vi "PopulateNist.vi"(11 "Path":path=path "") -> (3 "Array":string[](array[string]))   [LabVIEW 2014]
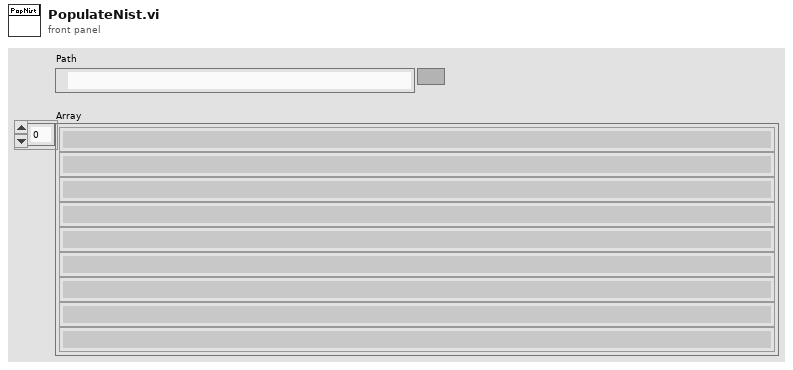
[diagram p1: front panel]
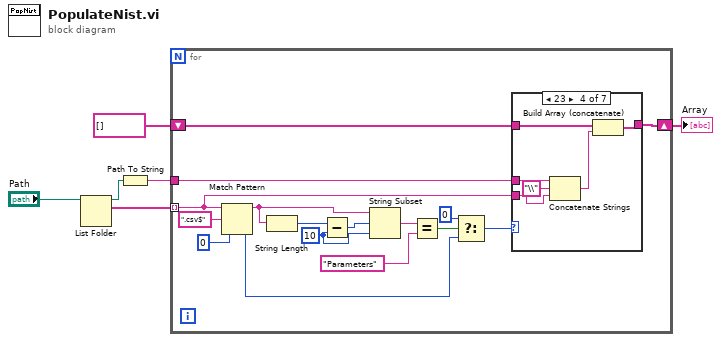
[diagram p0: block diagram]
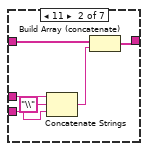
[diagram p3: hidden frame]
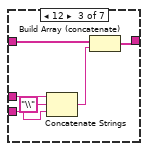
[diagram p4: hidden frame]
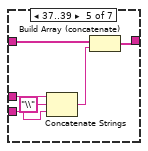
[diagram p5: hidden frame]
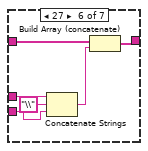
[diagram p6: hidden frame]
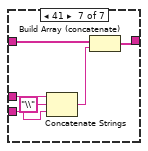
[diagram p7: hidden frame]
diagram:
  n1 = List Folder(path="Path") -> (path out=w4:path, filenames=w6:string[])  [unwired: 3 in, 2 out]
  n2 = Path To String(path=w4) -> (string=w3:string)
  n3 = for {
    tunnel: w6 -> [w20] mode=indexing
    tunnel: w3 -> [w19]
    shift-right: [w18] -> w1
    shift-left: string[] [] -> [w17]
    w14 = 10 ("y")
    n4 = Match Pattern(string=w20, regular expression=".csv$", offset (0)=0) -> (before substring=w7:string, offset past match=w10:i32)  [unwired: 2 out]
    n5 = String Length(string=w7) -> (length=w16:i32)
    n6 = Subtract(x=w16, y=w14) -> (x-y=w15:i32)
    n7 = String Subset(string=w7, offset (0)=w15, length (rest)=w14) -> (substring=w13:string)
    n8 = Equal?(x=w13, y="Parameters") -> (x = y?=w11:bool)
    n9 = Select(t=0, s=w11, f=w10) -> (s? t:f=w8:i32)
    n10 = case shown="23" w8 {
      tunnel: w20 -> [_ w24 w30 w36 w42 w48 w54]
      tunnel: w19 -> [_ w29 w35 w41 w47 w53 w59]
      tunnel: [w23 w26 w32 w38 w44 w50 w56] -> w18
      tunnel: w17 -> [w23 w28 w34 w40 w46 w52 w58]
      frame 0, Default {
      }
      frame 11 {
        n11 = Concatenate Strings(w29, "\\" ("string"), w24) -> (w27:string)
        n12 = Build Array (concatenate)(w28, w27) -> (w26:string[])
      }
      frame 12 {
        n13 = Concatenate Strings(w35, "\\" ("string"), w30) -> (w33:string)
        n14 = Build Array (concatenate)(w34, w33) -> (w32:string[])
      }
      frame 23 {
        n15 = Concatenate Strings(w41, "\\" ("string"), w36) -> (w39:string)
        n16 = Build Array (concatenate)(w40, w39) -> (w38:string[])
      }
      frame 37..39 {
        n17 = Concatenate Strings(w47, "\\" ("string"), w42) -> (w45:string)
        n18 = Build Array (concatenate)(w46, w45) -> (w44:string[])
      }
      frame 27 {
        n19 = Concatenate Strings(w53, "\\" ("string"), w48) -> (w51:string)
        n20 = Build Array (concatenate)(w52, w51) -> (w50:string[])
      }
      frame 41 {
        n21 = Concatenate Strings(w59, "\\" ("string"), w54) -> (w57:string)
        n22 = Build Array (concatenate)(w58, w57) -> (w56:string[])
      }
    }
  }
  "Array" <- w1
